vi "IsWired.vi"(6 "error in":errorcluster, 9 "Terminal in":refnum<class "Terminal.lvclass">) -> (0 "error out":errorcluster, 2 "wired":bool, 3 "Terminal out":refnum<class "Terminal.lvclass">)   [LabVIEW 2014, in "Raspberry Pi Compatible Compiler for LabVIEW.lvlib" / "Terminal.lvclass"]
uses:
  Terminal.lvclass
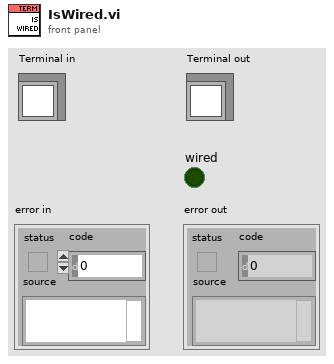
[diagram p1: front panel]
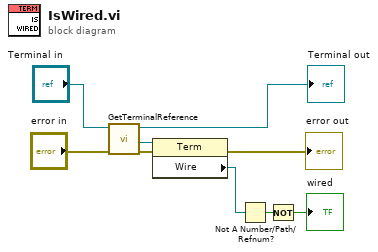
[diagram p0: block diagram]
diagram:
  n1 = call "GetTerminalReference.vi"("error in"="error in", "Terminal in"="Terminal in") -> ("error out"=w5:errorcluster, "reference"=w4:refnum<vi>, "Terminal out"=→"Terminal out":refnum<class "Terminal.lvclass">)  [unwired: 7 in]
  n2 = property class="Term"(reference=w4, error in=w5) -> (error out=→"error out":errorcluster, "Wire"=w8:refnum<vi>)  [unwired: 1 out]
  n3 = Not A Number/Path/Refnum?(number/path/refnum=w8) -> (NaN/Path/Refnum?=w7:bool)
  n4 = Not(x=w7) -> (.not. x?=→"wired":bool)
